vi "Detect oscillations.vi"(8 "Counter in":i32, 10 "Prev MC cmd":T1, 11 "Current MC cmd":T1) -> (0 "Counter out":i32)   [LabVIEW 2009]
uses:
  Remote Control/Motor Command.ctl
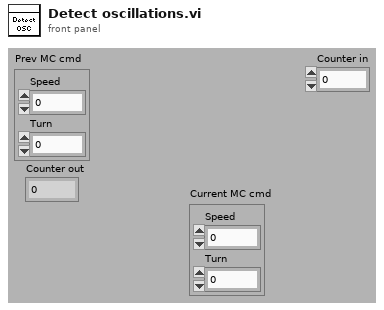
[diagram p1: front panel]
types:
  T1 = typedef "Motor Command.ctl" = cluster{"Speed":i16, "Turn":i16}
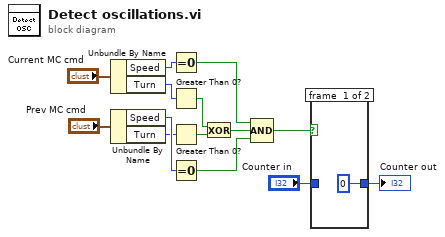
[diagram p0: block diagram]
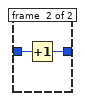
[diagram p2: hidden frame]
diagram:
  n1 = Unbundle By Name("Current MC cmd") -> ("Speed"=w13:i16, "Turn"=w10:i16)
  n2 = Unbundle By Name("Prev MC cmd") -> ("Speed"=w11:i16, "Turn"=w9:i16)
  n3 = Equal To 0?(x=w13) -> (x = 0?=w6:bool)
  n4 = Greater Than 0?(x=w10) -> (x > 0?=w8:bool)
  n5 = Greater Than 0?(x=w9) -> (x > 0?=w7:bool)
  n6 = Equal To 0?(x=w11) -> (x = 0?=w5:bool)
  n7 = Exclusive Or(1:w7, 2:w8) -> (0:w4:bool)
  n8 = Compound Arithmetic op=AND(w6, w4, w5) -> (w3:bool)
  n9 = case shown="False" w3 {
    tunnel: "Counter in" -> [_ w17]
    tunnel: [0 w16] -> w1
    frame #0 {
    }
    frame #1 {
      n10 = Increment(x=w17) -> (x+1=w16:i32)
    }
  }
  "Counter out" <- w1
